vi "通讯即时帮助.vi"(8 "error in (no error)":errorcluster caption="错误输入（无错误）", 11 "程序 输入":refnum<class "程序.lvclass">) -> (0 "error out":errorcluster caption="错误输出", 3 "程序 输出":refnum<class "程序.lvclass">)   [LabVIEW 2020, in "程序.lvclass"]
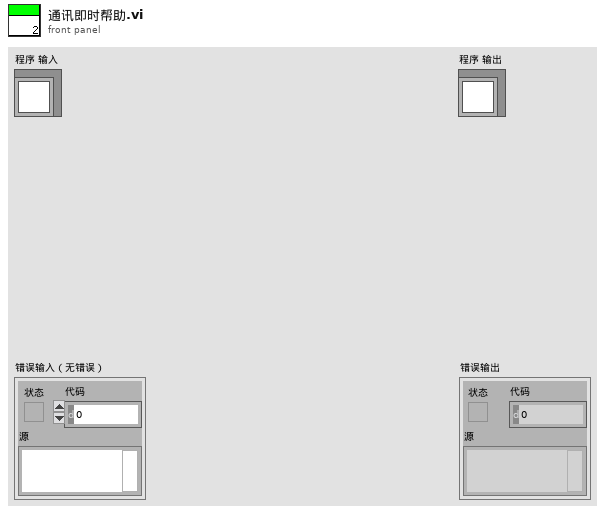
[diagram p1: front panel]
types:
  T1 = cluster{"名称":string, "关键字":string, "程序文本":string}
  T2 = enum32{"Invalid", "Standard", "Closed", "Hidden", "Minimized", "Maximized"}
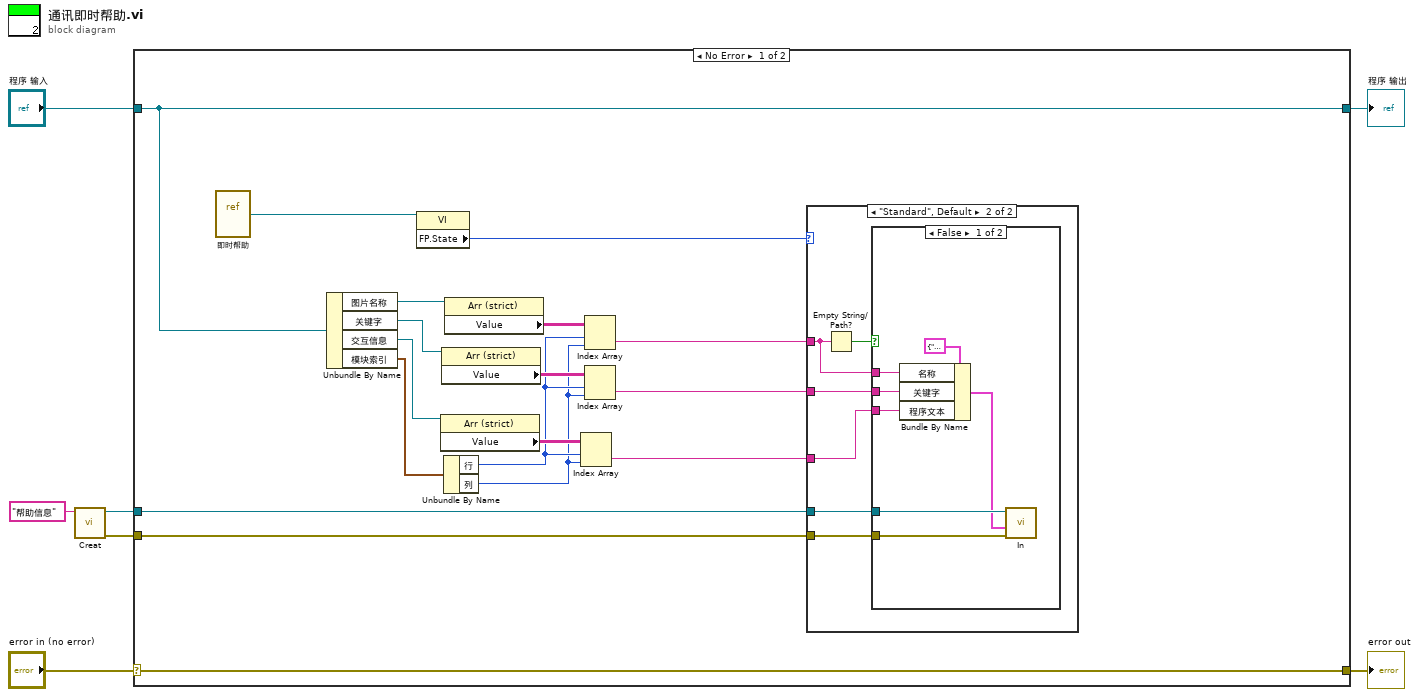
[diagram p0: block diagram]
diagram:
  n1 = call "Creat.vi"("名称"="帮助信息") -> ("错误输出"=w2:errorcluster, "队列输出"=w3:refnum<queue>)  [unwired: 9 in]
  n2 = case shown="No Error" "error in (no error)" {
    selector: "error in (no error)" -> [w25 w40]
    tunnel: [w25 w40] -> w6
    tunnel: [w22 w39] -> w4
    tunnel: "程序 输入" -> [w22 w39]
    tunnel: w3 -> [w24 _]
    tunnel: w2 -> [w23 _]
    frame No Error {
      n3 = vi-ref "即时帮助.vi"() -> (w9:refnum<vi>)
      n4 = Unbundle By Name(w22) -> ("图片名称"=w21:refnum<vi>, "关键字"=w15:refnum<vi>, "交互信息"=w20:refnum<vi>, "模块索引"=w17:cluster{"列":u32, "行":u32})
      n5 = property class="VI"(reference=w9) -> ("FP.State"=w8:T2)  [unwired: 1 in, 2 out]
      n6 = property class="Arr (strict)"(reference=w20) -> ("Value"=w18:string[][])  [unwired: 1 in, 2 out]
      n7 = property class="Arr (strict)"(reference=w15) -> ("Value"=w14:string[][])  [unwired: 1 in, 2 out]
      n8 = Unbundle By Name(w17) -> ("行"=w13:u32, "列"=w12:u32)
      n9 = property class="Arr (strict)"(reference=w21) -> ("Value"=w19:string[][])  [unwired: 1 in, 2 out]
      n10 = Index Array(array=w18, index (row)=w13, index (col)=w12) -> (element=w16:string)
      n11 = Index Array(array=w19, index (row)=w13, index (col)=w12) -> (element=w10:string)
      n12 = Index Array(array=w14, index (row)=w13, index (col)=w12) -> (element=w11:string)
      n13 = case shown="\"Standard\", Default" w8 {
        tunnel: w24 -> [_ w31]
        tunnel: w23 -> [_ w30]
        tunnel: w16 -> [_ w29]
        tunnel: w11 -> [_ w28]
        tunnel: w10 -> [_ w26]
        frame "Invalid", "Closed" {
        }
        frame "Standard", Default {
          n14 = Empty String/Path?(string/path=w26) -> (empty?=w27:bool)
          n15 = case shown="False" w27 {
            tunnel: w31 -> [w38 _]
            tunnel: w30 -> [w37 _]
            tunnel: w26 -> [w35 _]
            tunnel: w29 -> [w34 _]
            tunnel: w28 -> [w33 _]
            frame False {
              n16 = Bundle By Name(cluster=T1 {"名称"="", "关键字"="", "程序文本"=""}, "名称"=w35, "关键字"=w33, "程序文本"=w34) -> (w32:T1)
              n17 = call "In.vi"("错误输入"=w37, "数据"=w32, "队列"=w38) -> ()  [unwired: 7 in, 2 out]
            }
            frame True {
            }
          }
        }
      }
    }
    frame Error {
    }
  }
  "error out" <- w6
  "程序 输出" <- w4
